vi "OpenG Array filter - Template.vi"() -> ()   [LabVIEW 2018]
panel:
  out "filtered item indices":i32[](array[numeric])
  out "filtered array":variant[](array[variant])
  in  "items to filter":variant[](array[variant])
  in  "Array Input":variant[](array[variant])
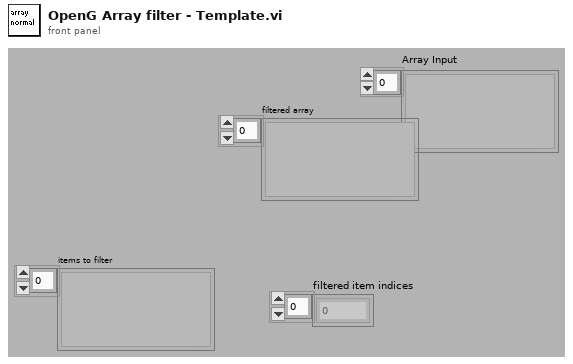
[diagram p1: front panel]
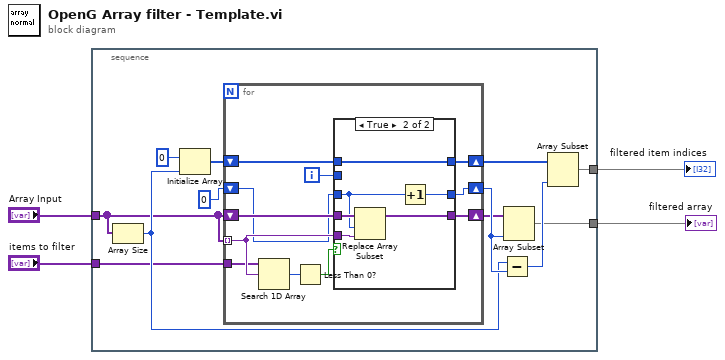
[diagram p0: block diagram]
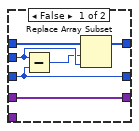
[diagram p2: hidden frame]
diagram:
  n1 = stacked-sequence {
    tunnel: "items to filter" -> [w7]
    tunnel: [w5] -> w3
    tunnel: "Array Input" -> [w8]
    tunnel: [w6] -> w1
    frame #0 {
      n2 = Array Size(array=w8) -> (size(s)=w13:i32)
      n3 = Initialize Array(0 ("Numeric"), w13) -> (w12:i32[])
      n4 = for {
        tunnel: w8 -> [w24] mode=indexing
        shift-right: [w25] -> w10
        shift-left: w8 -> [w27]
        shift-right: [w22] -> w15
        shift-left: 0 -> [w23]
        shift-right: [w19] -> w14
        shift-left: w12 -> [w20]
        tunnel: w7 -> [w18]
        i -> [w17]
        n5 = Search 1D Array(1D array=w18, element=w24) -> (index of element=w21:i32)  [unwired: 1 out]
        n6 = Less Than 0?(x=w21) -> (x < 0?=w26:bool)
        n7 = case shown="True" w26 {
          tunnel: w27 -> [w33 w39]
          tunnel: [w33 w38] -> w25
          tunnel: w24 -> [_ w37]
          tunnel: w23 -> [w29 w35]
          tunnel: [w29 w36] -> w22
          tunnel: w20 -> [w32 w34]
          tunnel: [w31 w34] -> w19
          tunnel: w17 -> [w30 _]
          frame False {
            n8 = Subtract(x=w30, y=w29) -> (x-y=w28:i32)
            n9 = Replace Array Subset(array=w32, new element=w30, index=w28) -> (w31:i32[])
          }
          frame True {
            n10 = Replace Array Subset(array=w39, new element=w37, index=w35) -> (w38:variant[])
            n11 = Increment(x=w35) -> (x+1=w36:i32)
          }
        }
      }
      n12 = Subtract(x=w13, y=w15) -> (x-y=w16:i32)
      n13 = Array Subset(array=w10, length=w15) -> (w6:variant[])  [unwired: 1 in]
      n14 = Array Subset(array=w14, length=w16) -> (w5:i32[])  [unwired: 1 in]
    }
  }
  "filtered array" <- w1
  "filtered item indices" <- w3
